vi "Read Turbo SM State.vi"(8 "error in (no error)":errorcluster, 9 "State Timeout (Inf)":dbl=inf, 10 "Reinit Timer (F)":bool, 11 "Turbo in":refnum<class "Turbo.lvclass">) -> (0 "error out":errorcluster, 1 "Sample Transfer State":string, 2 "Turbo State":T5=enum."Idle", 3 "Turbo out":refnum<class "Turbo.lvclass">, 4 "Timeout?":bool, 5 "Turbo Pump State":T4 {"Gauge 1 Reading" format="%.2e"; "Pump Power (W)" format="%.1f"; "Pump Speed (%)" format="%.1f"}, 6 "State Timeout":dbl)   [LabVIEW 2015, in "cRIO-Carbondioxide.lvlib" / "CO2-Actor.lvlib" / "Turbo.lvclass"]
uses:
  Turbo.lvclass
  Turbo State Enumerator.ctl
  <instrlib>/BOC Edwards TIC/Turbo Instrument Controller.llb/Type Def - Pump State.ctl
  <instrlib>/BOC Edwards TIC/Turbo Instrument Controller.llb/Type Def - Alert ID.ctl
  <instrlib>/BOC Edwards TIC/Turbo Instrument Controller.llb/Type Def - Priority.ctl
  Turbo.lvclass/Turbo.ctl
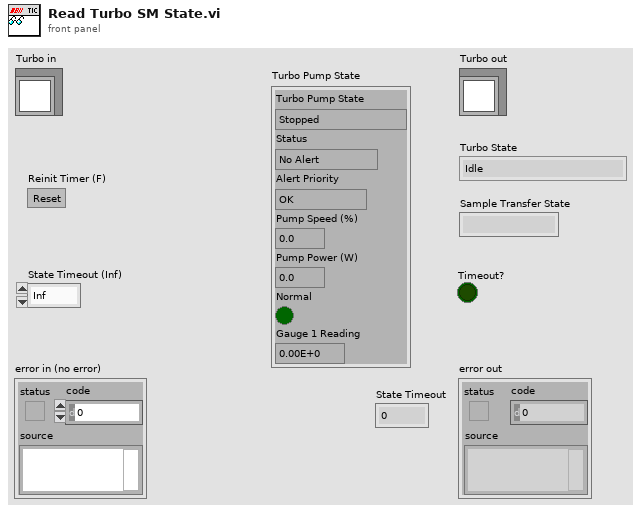
[diagram p1: front panel]
types:
  T1 = typedef "Type Def - Pump State.ctl" = enum16{"Stopped", "Starting Delay", "Stopping Short Delay", "Stopping Normal Delay", "Running", "Accelerating", "Fault Braking", "Braking"}
  T2 = typedef "Type Def - Alert ID.ctl" = enum16{"No Alert", "ADC Fault", "ADC Not Ready", "Over Range", "Under Range", "ADC Invalid", "No Gauge", "Unknown", "Not Supported", "New ID", "Ion EM Timeout", "Not Struck", "Filament Fail", "Mag Fail", "Striker Fail", "Cal Error", "Initialising", "Emission Error", "Over Pressure", "ASG Can't Zero", "Ramp Up Timeout", "Droop Timeout", "Run Hours High", "SC Interlock", "ID Volts Error", "Serial ID Fail", "Upload Active", "DX Fault", "Temp Alert", "SYSI Inhibit", "Ext Inhibit", "Temp Inhibit", "No Reading", "No Message", "NOV Failure", "ULoad Timeout", "DLoad Failed", "No Tube"}
  T3 = typedef "Type Def - Priority.ctl" = enum16{"OK", "Warning", "Alarm"}
  T4 = cluster{"Turbo Pump State":T1, "Status":T2, "Alert Priority":T3, "Pump Speed (%)":dbl, "Pump Power (W)":dbl, "Normal":bool, "Gauge 1 Reading":dbl}
  T5 = typedef "cRIO-Carbondioxide.lvlib/CO2-Actor.lvlib/Turbo.lvclass/Turbo State Enumerator.ctl" = enum16{"Undefined", "Error", "Abort", "Idle", "Initialize", "Start FV Pump", "Wait on FV Gauge", "Start Turbo", "Running", "Stop"}
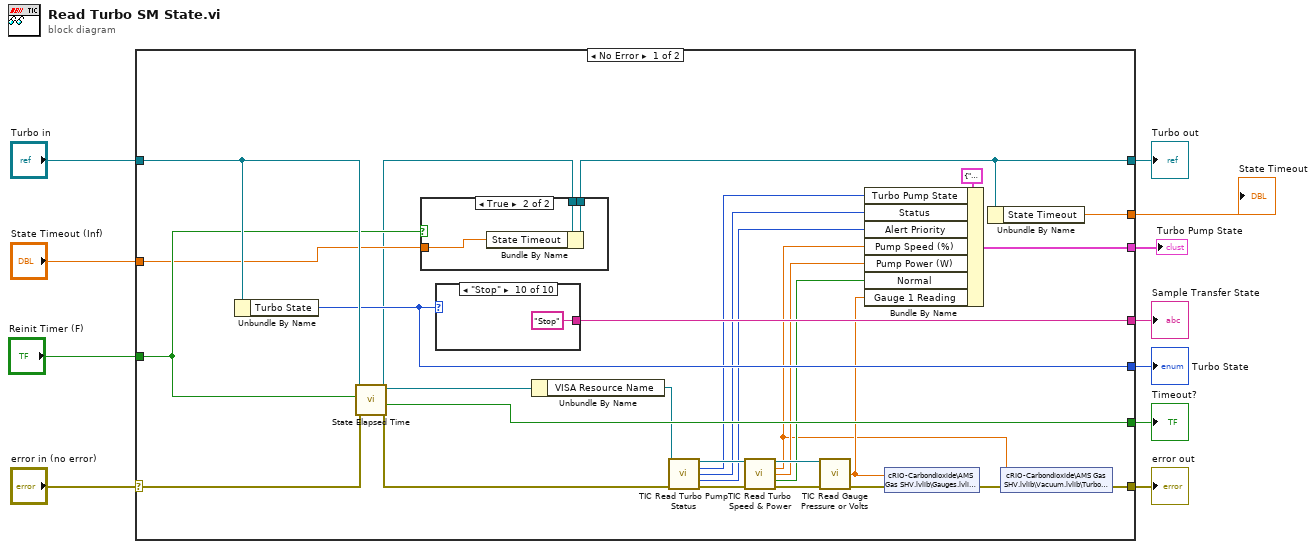
[diagram p0: block diagram]
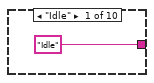
[diagram p3: hidden frame]
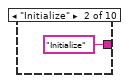
[diagram p4: hidden frame]
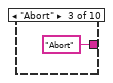
[diagram p5: hidden frame]
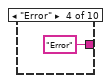
[diagram p6: hidden frame]
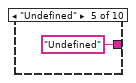
[diagram p7: hidden frame]
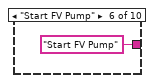
[diagram p8: hidden frame]
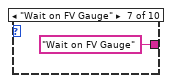
[diagram p9: hidden frame]
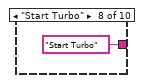
[diagram p10: hidden frame]
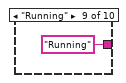
[diagram p11: hidden frame]
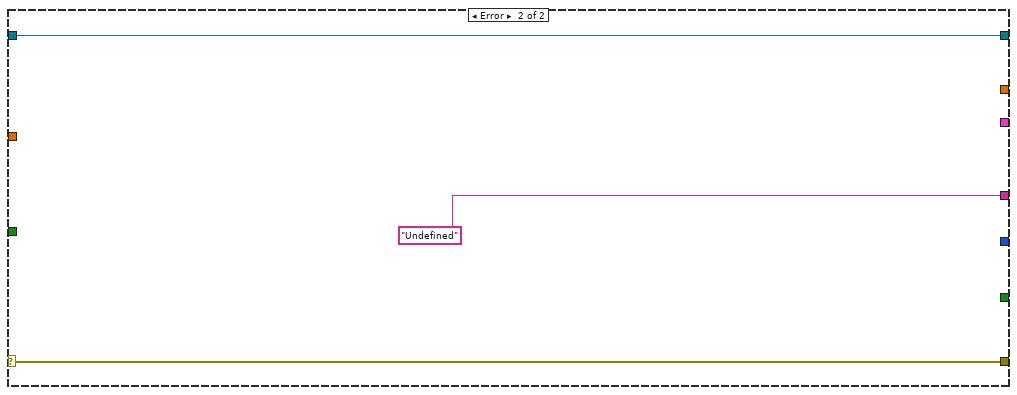
[diagram p12: hidden frame]
diagram:
  n1 = case shown="No Error" "error in (no error)" {
    selector: "error in (no error)" -> [w36 w55]
    tunnel: [w14 w55] -> w10
    tunnel: [w13 w56] -> w8
    tunnel: "Turbo in" -> [w37 w56]
    tunnel: [w33 _] -> w7
    tunnel: [w39 "Undefined"] -> w6
    tunnel: [w38 _] -> w5
    tunnel: "Reinit Timer (F)" -> [w35 _]
    tunnel: "State Timeout (Inf)" -> [w34 _]
    tunnel: [w23 _] -> w2
    tunnel: [w12 _] -> w1
    frame No Error {
      n2 = Unbundle By Name(w37) -> ("Turbo State"=w33:T5)
      n3 = call "State Elapsed Time.vi"("error in (no error)"=w36, "Reset (F)"=w35, "Turbo in"=w37) -> ("error out"=w32:errorcluster, "State Timeout?"=w38:bool, "Turbo out"=w29:refnum<class "Turbo.lvclass">)  [unwired: 5 in, 1 out]
      n4 = case shown="True" w35 {
        tunnel: w29 -> [w40 w43]
        tunnel: [w40 w42] -> w13
        tunnel: w34 -> [_ w41]
        frame False {
        }
        frame True {
          n5 = Bundle By Name(cluster=w43, "State Timeout"=w41) -> (w42:refnum<class "Turbo.lvclass">)
        }
      }
      n6 = case shown="\"Stop\"" w33 {
        tunnel: ["Idle" "Initialize" "Abort" "Error" "Undefined" "Start FV Pump" "Wait on FV Gauge" "Start Turbo" "Running" "Stop"] -> w39
        frame "Idle" {
        }
        frame "Initialize" {
        }
        frame "Abort" {
        }
        frame "Error" {
        }
        frame "Undefined" {
        }
        frame "Start FV Pump" {
        }
        frame "Wait on FV Gauge" {
        }
        frame "Start Turbo" {
        }
        frame "Running" {
        }
        frame "Stop" {
        }
      }
      n7 = Unbundle By Name(w29) -> ("VISA Resource Name"=w28:refnum<visa-resource-name>)
      n8 = call <instrlib>:"TIC Read Turbo Pump Status.vi"("VISA Resource Name"=w28, "error in (no error)"=w32) -> ("VISA session (Dup)"=w27:refnum<visa-resource-name>, "Turbo Pump State"=w24:T1, "Status"=w22:T2, "Alert Priority"=w21:T3, "error out"=w31:errorcluster)  [unwired: 9 in]
      n9 = call <instrlib>:"TIC Read Turbo Speed & Power.vi"("VISA Resource Name"=w27, "error in (no error)"=w31) -> ("VISA session (Dup)"=w26:refnum<visa-resource-name>, "Pump Speed (%)"=w15:dbl, "Pump Power (W)"=w20:dbl, "Normal"=w19:bool, "error out"=w30:errorcluster)  [unwired: 9 in]
      n10 = call <instrlib>:"TIC Read Gauge Pressure or Volts.vi"("VISA Session In"=w26, "error in (no error)"=w30) -> ("Reading"=w17:dbl, "error out"=w18:errorcluster)  [unwired: 9 in, 3 out]
      n11 = Bundle By Name(cluster=T4 {"Turbo Pump State"=enum."Stopped", "Status"=enum."No Alert", "Alert Priority"=enum."OK", "Pump Speed (%)"=0.0, "Pump Power (W)"=0.0, "Normal"=FALSE, "Gauge 1 Reading"=0.0} ("Turbo Pump State"), "Turbo Pump State"=w24, "Status"=w22, "Alert Priority"=w21, "Pump Speed (%)"=w15, "Pump Power (W)"=w20, "Normal"=w19, "Gauge 1 Reading"=w17) -> (w23:T4)
      n12 = shared-variable "cRIO-Carbondioxide\\AMS Gas SHV.lvlib\\Gauges.lvlib\\FV Gauge"(w17, error in=w18) -> (error out=w16:errorcluster)
      n13 = Unbundle By Name(w13) -> ("State Timeout"=w12:dbl)
      n14 = shared-variable "cRIO-Carbondioxide\\AMS Gas SHV.lvlib\\Vacuum.lvlib\\Turbo Speed"(w15, error in=w16) -> (error out=w14:errorcluster)
    }
    frame Error {
    }
  }
  "error out" <- w10
  "Turbo out" <- w8
  "Turbo State" <- w7
  "Sample Transfer State" <- w6
  "Timeout?" <- w5
  "Turbo Pump State" <- w2
  "State Timeout" <- w1
